vi "tank.vi"() -> ()   [LabVIEW 2018]
panel:
  out "Tank":dbl(slide) scale=0.0..10.0
  in  "Numeric":dbl
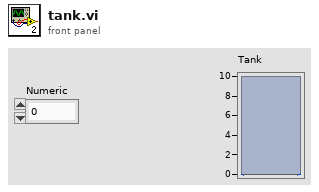
[diagram p1: front panel]
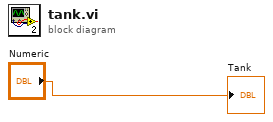
[diagram p0: block diagram]
diagram:
  "Tank" <- "Numeric"
